vi "Freq_to_FTW.vi"(1 "Frequency (MHz)":dbl, 12 "Channel Parameters":T1 {"Ref Clock Rate [MHz]" min=0.0}) -> (21 "FTW (32bit)":u32)   [LabVIEW 2013, in "DDS.lvlib"]
uses:
  DDS.lvlib
  Controls/DDS Channel Parameters.ctl
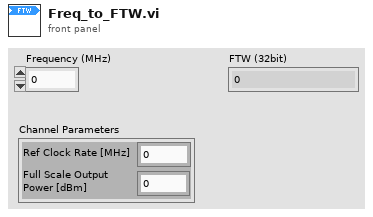
[diagram p1: front panel]
types:
  T1 = typedef "DDS.lvlib/DDS Channel Parameters.ctl" = cluster{"Ref Clock Rate [MHz]":dbl, "Full Scale Output\nPower [dBm]":dbl}
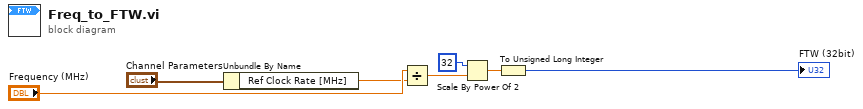
[diagram p0: block diagram]
diagram:
  n1 = Unbundle By Name("Channel Parameters") -> ("Ref Clock Rate [MHz]"=w4:dbl)
  n2 = Divide(x="Frequency (MHz)", y=w4) -> (x/y=w1:dbl)
  n3 = Scale By Power Of 2(n=32 ("x"), x=w1) -> (x*2^n=w3:dbl)
  n4 = To Unsigned Long Integer(number=w3) -> (unsigned 32bit integer=→"FTW (32bit)":u32)
